vi "About Panther Dashboard.vi"(8 "error in":errorcluster) -> (0 "error out":errorcluster)   [LabVIEW 2019, in "Panther Dashboard.lvlib"]
uses:
  Panther Dashboard.lvlib
  <vilib>/Platform/browser.llb/Open URL in Default Browser (string).vi
panel:
  out "Title":string
  in  "Website":bool
  in  "About DQMH":bool
  # "Developed and maintained by \nPantherLAB"
  # "Main Contributor- Developer:\n\n» Enrique Noé Arias\n\nBrainstorming & Code Reviews (Alphabetical order):\n\n» Matthias Baudot\n» Fabiola De La Cueva\n» Christopher Farmer\n» Cyril Gambini\n» Joerg Hampel\n» Olivier Jourdan\n» Casey May\n» Cesar Muñoz\n» Darren Nattinger\n» Luis Orozco\n» Sam Taggart\n» Diego Torres"
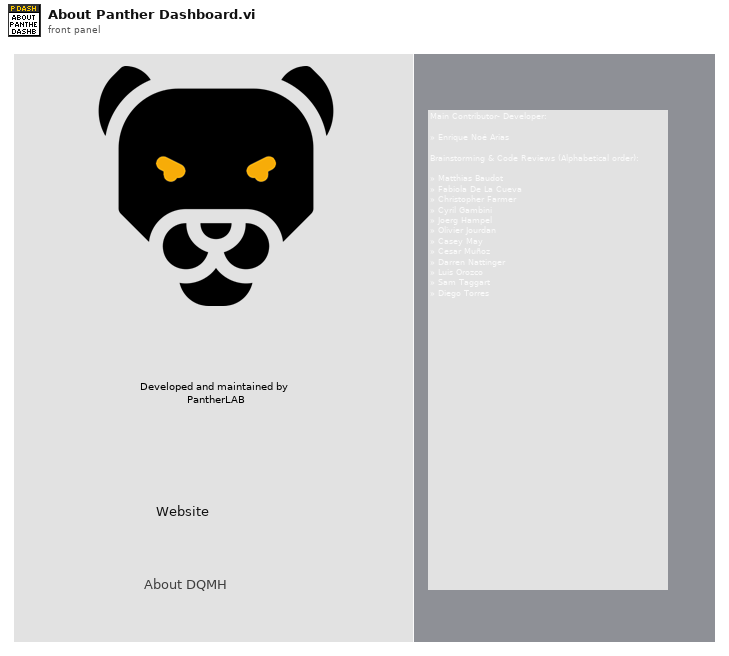
[diagram p1: front panel]
types:
  T1 = cluster{"Major":u16, "Minor":u16, "Fix":u16, "Build":u16}
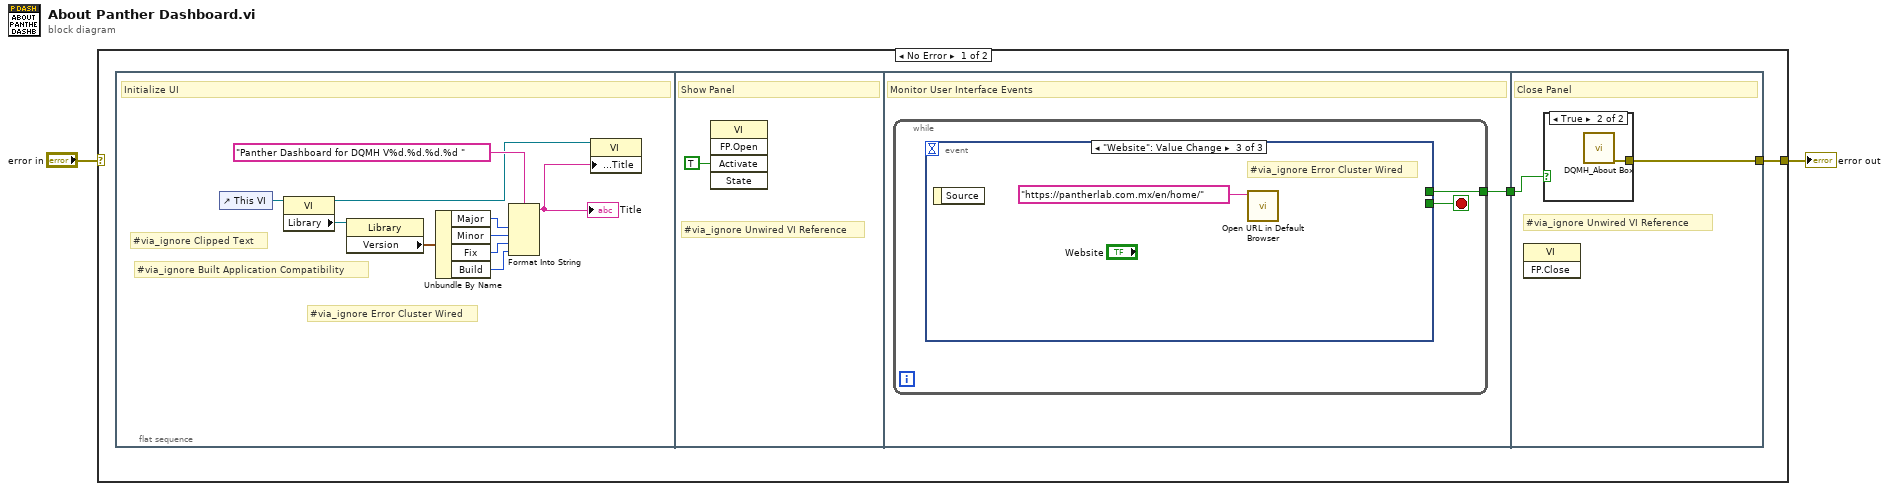
[diagram p0: block diagram]
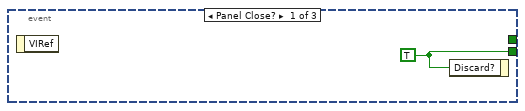
[diagram p2: hidden frame]
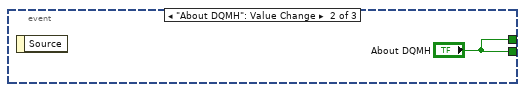
[diagram p3: hidden frame]
diagram:
  n1 = case shown="No Error" "error in" {
    selector: "error in" -> [_ w25]
    tunnel: [w4 w25] -> w1
    frame No Error {
      n2 = flat-sequence {
        tunnel: [w16] -> w3
        tunnel: w3 -> [w22]
        tunnel: [w23] -> w4
        frame #0 {
          # "#via_ignore Clipped Text"
          # "#via_ignore Built Application Compatibility"
          # "#via_ignore Error Cluster Wired"
          # "Initialize UI"
          n3 = control-ref of="This VI"() -> (w13:refnum<vi>)
          n4 = property class="VI"(reference=w13) -> (reference out=w6:refnum<vi>, "Library"=w12:refnum<vi>)  [unwired: 1 in, 1 out]
          n5 = property class="Library"(reference=w12) -> ("Version"=w11:T1)  [unwired: 1 in, 2 out]
          n6 = Unbundle By Name(w11) -> ("Major"=w10:u16, "Minor"=w9:u16, "Fix"=w8:u16, "Build"=w7:u16)
          n7 = Format Into String(format string="Panther Dashboard for DQMH V%d.%d.%d.%d " ("String"), w10, w9, w8, w7) -> (resulting string=w5:string)  [unwired: 2 in, 1 out]
          "Title" <- w5
          n8 = property class="VI"(reference=w6, "Front Panel.Title"=w5) -> ()  [unwired: 1 in, 2 out]
        }
        frame #1 {
          # "#via_ignore Unwired VI Reference"
          # "Show Panel"
          n9 = invoke class="VI" method="FP.Open"("Activate"=TRUE ("Activate?")) -> ()  [unwired: 4 in, 5 out]
        }
        frame #2 {
          # "Monitor User Interface Events"
          n10 = while {
            tunnel: [w17] -> w16
            stop <- w18 stop-if-true
            n11 = event shown="[2] \"Website\": Value Change" {
              selector: _ -> [_ _ _]
              dyn-events: _ -> [_ _ _]
              timeout: _ -> [_ _ _]
              tunnel: [w19 "About DQMH" _] -> w18
              tunnel: [_ "About DQMH" _] -> w17
              event Panel Close? {
                w19 = TRUE ("Discard?")
                n12 = event-data() -> ()  [unwired: 1 in, 1 out]
                n13 = event-data("Discard?"=w19) -> ()  [unwired: 1 in, 1 out]
              }
              event "About DQMH": Value Change {
                n14 = event-data() -> ()  [unwired: 1 in, 1 out]
              }
              event "Website": Value Change {
                # "#via_ignore Error Cluster Wired"
                n15 = event-data() -> ()  [unwired: 1 in, 1 out]
                n16 = call-poly <vilib>:"Open URL in Default Browser.vi"("URL"="https://pantherlab.com.mx/en/home/") -> ()  [unwired: 5 in, 2 out]
              }
            }
          }
        }
        frame #3 {
          # "#via_ignore Unwired VI Reference"
          # "Close Panel"
          n17 = invoke class="VI" method="FP.Close"() -> ()  [unwired: 3 in, 3 out]
          n18 = case shown="True" w22 {
            tunnel: [_ w24] -> w23
            frame False {
            }
            frame True {
              n19 = call <vilib>:"DQMH_About Box.vi"() -> ("error out"=w24:errorcluster)  [unwired: 11 in]
            }
          }
        }
      }
    }
    frame Error {
    }
  }
  "error out" <- w1
